vi "Entry.vi"(8 "error in (no error)":errorcluster, 11 "State Machine in":refnum<class "State Machine.lvclass">) -> (0 "error out":errorcluster, 3 "State Machine out":refnum<class "State Machine.lvclass">)   [LabVIEW 2024, in "State Pattern Actor.lvlib" / "State Machine.lvlib" / "State Machine.lvclass"]
uses:
  State Machine.lvclass
  State Machine.lvclass/State Machine.ctl
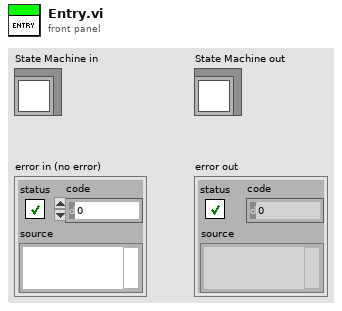
[diagram p1: front panel]
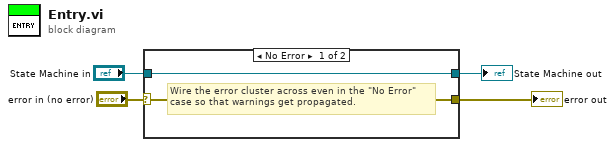
[diagram p0: block diagram]
diagram:
  n1 = case shown="No Error" "error in (no error)" {
    selector: "error in (no error)" -> [w5 w8]
    tunnel: [w5 w8] -> w3
    tunnel: [w6 w7] -> w1
    tunnel: "State Machine in" -> [w6 w7]
    frame No Error {
      # "Wire the error cluster across even in the \"No Error\"\ncase so that warnings get propagated."
    }
    frame Error {
    }
  }
  "error out" <- w3
  "State Machine out" <- w1
